vi "Test JSON Conversion.vi"() -> ()   [LabVIEW 2014]
uses:
  reusable/CRDS/Data/Cell/CRDS Cell Data.lvclass
  reusable/CRDS/Cell/extParam Ctl.ctl
  reusable/CRDS/Cell/hkParam Ctl.ctl
  reusable/PAS/Data/Cell/PAS Cell Data.lvclass
  reusable/CRDS/Data/Cell/CRDS Cell Data.lvclass/CRDS Cell Data.ctl
  reusable/PAS/Data/Cell/PAS Cell Data.lvclass/PAS Cell Data.ctl
  reusable/PAS/Data/Cell/Read fit data.vi
  reusable/PAS/Data/Cell/Read IAbackground.vi
  reusable/CRDS/Data/Cell/Read extParam.vi
  reusable/CRDS/Data/Cell/Read Allan Variances.vi
  reusable/PAS/Data/Cell/Read derived.vi
  reusable/PAS/Data/Cell/Read Fitted Data.vi
  reusable/PAS/Data/Cell/Read freqData.vi
  reusable/PAS/Data/Cell/Read timeData.vi
  reusable/PAS/Data/Cell/Read lasDiodeData.vi
  reusable/CRDS/Data/Cell/Read hkParam.vi
  reusable/CRDS/Data/Cell/Read Ringdowns.vi
  reusable/CRDS/CRDS Lib.lvlib
  <vilib>/measure/NI_MABase.lvlib
panel:
  out "Numeric Control":u32
  out "JSONData":string
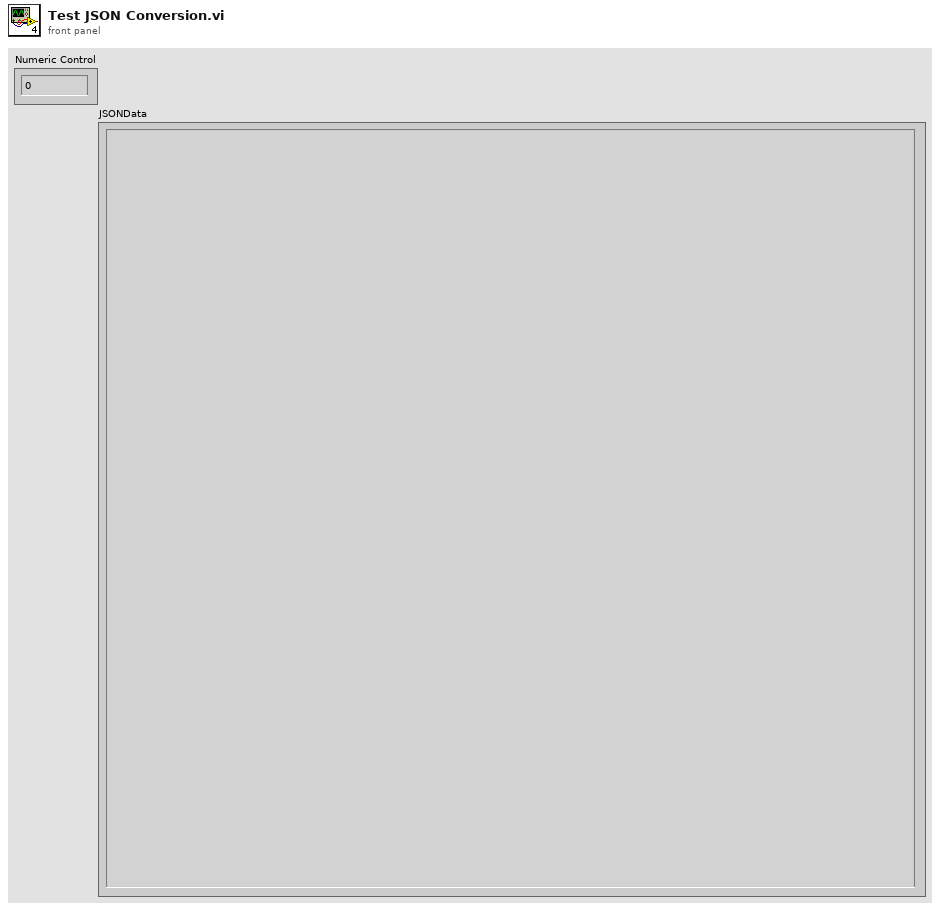
[diagram p1: front panel]
types:
  T1 = enum16{"Sine Wave", "Triangle Wave", "Square Wave", "Sawtooth Wave"}
  T2 = typedef "CRDS Lib.lvlib/extParam Ctl.ctl" = cluster{"Tau":sgl, "Tau0cor":sgl, "ext":sgl, "extCorr":sgl, "stdevTau":sgl, "eTau":sgl, "taucorr":sgl, "Tau0":sgl, "max":sgl}
  T3 = typedef "hkParam Ctl.ctl" = cluster{"rhDilFac":sgl, "Q":sgl, "Tmean":sgl, "extDilFac":sgl, "rhCell":sgl, "P":sgl, "T":sgl}
  T4 = cluster{"Time":dbl, "CellData":cluster{"extParam":T2, "hk":T3, "RDs":i16[][], "Data Access:Allan Variances":cluster{"iTime":sgl[], "stdev":sgl[]}}[]}
  T5 = cluster{"extParam":T2, "hk":T3, "RDs":i16[][], "Data Access:Allan Variances":cluster{"iTime":sgl[], "stdev":sgl[]}}
  T6 = typedef "extParam Ctl.ctl" = cluster{"Tau":sgl, "Tau0cor":sgl, "ext":sgl, "extCorr":sgl, "stdevTau":sgl, "eTau":sgl, "taucorr":sgl, "Tau0":sgl, "max":sgl}
  T7 = cluster{"f0":sgl, "IA":sgl, "Q":sgl, "max":dbl[], "noiseLim":dbl, "ext":dbl}
  T8 = typedef "NI_Matrix.lvlib/RealMatrix.ctl" = dbl[][]
  T9 = cluster{"Accessors:derived":cluster{"f0":sgl, "IA":sgl, "Q":sgl, "max":dbl[], "noiseLim":dbl, "ext":dbl}, "Accessors:fit data":cluster{"parameters":dbl[], "covariance":T8}, "Accessors:IAbackground":dbl}
  T10 = cluster{"extParam":T2, "hk":T3, "RDs":i16[][], "Data Access:Allan Variances":cluster{"iTime":sgl[], "stdev":sgl[]}}[]
  T11 = cluster{dbl, cluster{"Accessors:derived":cluster{"f0":sgl, "IA":sgl, "Q":sgl, "max":dbl[], "noiseLim":dbl, "ext":dbl}, "Accessors:fit data":cluster{"parameters":dbl[], "covariance":T8}, "Accessors:IAbackground":dbl}[], cluster{"Y":dbl[], "dt":dbl}[], cluster{"Y":dbl[], "dt":dbl}[], cluster{"Y":dbl[], "dt":dbl}[]}
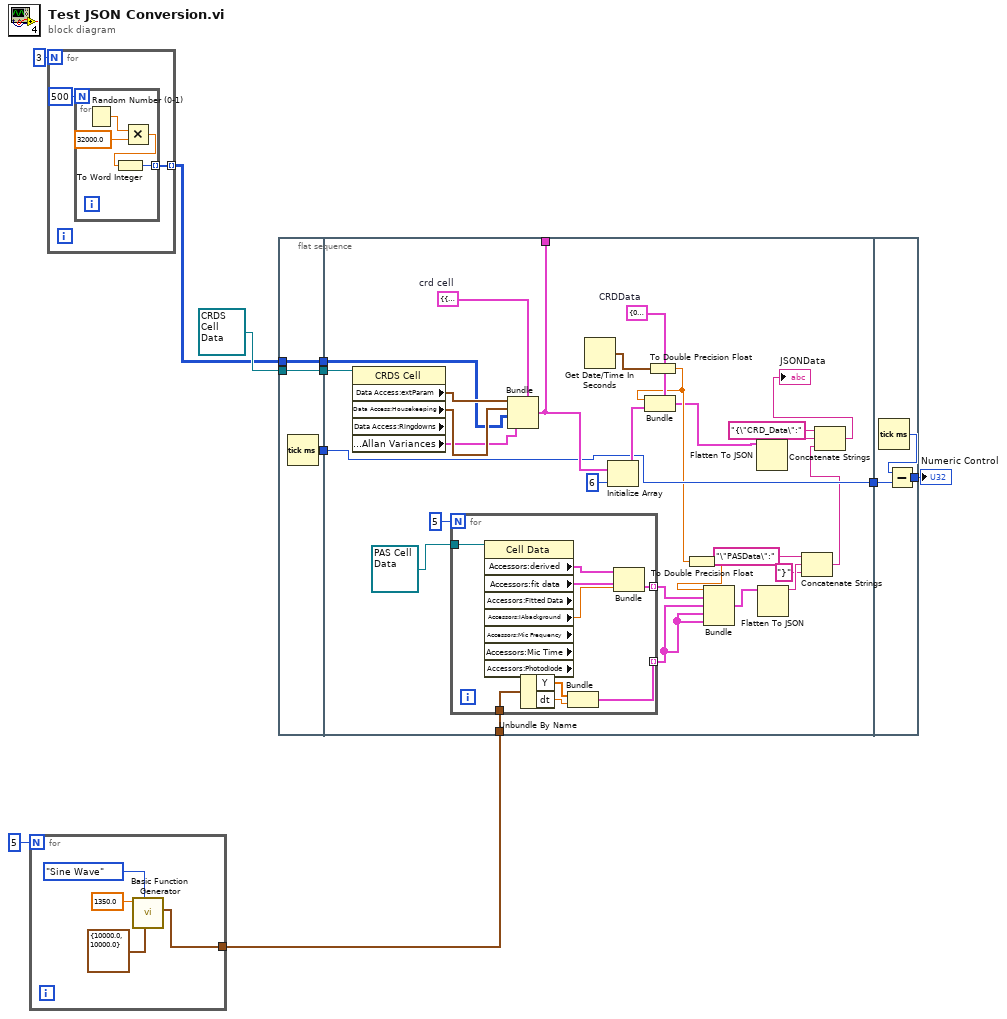
[diagram p0: block diagram]
diagram:
  n1 = for {
    N: 5 -> [_]
    tunnel: [w11] -> w1
    n2 = call <vilib>:"Basic Function Generator.vi"("sampling info"=cluster{"Fs":dbl, "#s":dbl} {"Fs"=10000.0, "#s"=10000.0}, "signal type"=T1."Sine Wave", "frequency"=1350.0) -> ("signal out"=w11:waveform(dbl))  [unwired: 6 in, 2 out]
  }
  n3 = for {
    N: 3 -> [_]
    tunnel: [w15] -> w8 mode=indexing
    n4 = for {
      N: 500 -> [_]
      tunnel: [w17] -> w15 mode=indexing
      n5 = Random Number (0-1)() -> (number: 0 to 1=w20:dbl)
      n6 = Multiply(x=w20, y=32000.0) -> (x*y=w18:dbl)
      n7 = To Word Integer(number=w18) -> (16bit integer=w17:i16)
    }
  }
  n8 = flat-sequence {
    tunnel: w8 -> [w22]
    tunnel: refnum<class "CRDS Cell Data.lvclass"> refnum ("CRDS Cell") -> [w23]
    tunnel: [w23] -> w7
    tunnel: [w22] -> w6
    tunnel: [w21] -> w4
    tunnel: [w45] -> _
    tunnel: w7 -> [w51]
    tunnel: w6 -> [w46]
    tunnel: [w41] -> w5
    tunnel: w4 -> [w41]
    tunnel: w1 -> [w36]
    tunnel: w5 -> [w62]
    tunnel: [w61] -> w3
    frame #0 {
      n9 = Tick Count (ms)() -> (millisecond timer value=w21:u32)
    }
    frame #1 {
      w40 = T4 {"Time"=0.0, "CellData"=[]}  # CRDData
      w47 = T5 {"extParam"={"Tau"=0.0, "Tau0cor"=0.0, "ext"=0.0, "extCorr"=0.0, "stdevTau"=0.0, "eTau"=0.0, "taucorr"=0.0, "Tau0"=0.0, "max"=0.0}, "hk"={"rhDilFac"=0.0, "Q"=0.0, "Tmean"=0.0, "extDilFac"=0.0, "rhCell"=0.0, "P"=0.0, "T"=0.0}, "RDs"=[], "Data Access:Allan Variances"={"iTime"=[], "stdev"=[]}}  # crd cell
      n10 = property class="CRDS Cell" props=["Data Access:extParam", "Data Access:Housekeeping", "Data Access:Ringdowns", "Data Access:Allan Variances"](reference=w51) -> ("Data Access:extParam"=w50:T6, "Data Access:Housekeeping"=w49:T3, "Data Access:Allan Variances"=w48:cluster{"iTime":i32[], sgl[]})  [unwired: 1 in, 3 out]
      n11 = for {
        N: 5 -> [_]
        tunnel: refnum<class "PAS Cell Data.lvclass"> refnum ("Cell Data") -> [w60]
        tunnel: w36 -> [w53]
        tunnel: [w56] -> w35 mode=indexing
        tunnel: [w52] -> w34 mode=indexing
        n12 = property class="Cell Data" props=["Accessors:derived", "Accessors:fit data", "Accessors:Fitted Data", "Accessors:IAbackground", "Accessors:Mic Frequency", "Accessors:Mic Time", "Accessors:Photodiode"](reference=w60) -> ("Accessors:derived"=w59:T7, "Accessors:fit data"=w58:cluster{"parameters":dbl[], "covariance":T8}, "Accessors:IAbackground"=w57:dbl)  [unwired: 1 in, 6 out]
        n13 = Unbundle By Name(w53) -> ("Y"=w54:dbl[], "dt"=w55:dbl)
        n14 = Bundle("Y"=w54, "dt"=w55) -> (w52:cluster{"Y":dbl[], "dt":dbl})  [unwired: 1 in]
        n15 = Bundle("Accessors:derived"=w59, "Accessors:fit data"=w58, "Accessors:IAbackground"=w57) -> (w56:T9)  [unwired: 1 in]
      }
      n16 = Bundle(cluster=w47, "extParam"=w50, "hk"=w49, "RDs"=w46, "Data Access:Allan Variances"=w48) -> (w45:T5)
      n17 = Get Date/Time In Seconds() -> (seconds since 1Jan1904=w43:timestamp)
      n18 = Initialize Array(w45, 6 ("dimension size")) -> (w42:T10)
      n19 = To Double Precision Float(number=w43) -> (double precision float=w38:dbl)
      n20 = Bundle(cluster=w40, "Time"=w38, "CellData"=w42) -> (w33:T4)
      n21 = To Double Precision Float(number=w38) -> (double precision float=w37:dbl)
      n22 = Bundle(w37, w35, w34, w34, w34) -> (w32:T11)  [unwired: 1 in]
      n23 = Flatten To JSON(anything=w33) -> (JSON string=w30:string)  [unwired: 2 in, 1 out]
      n24 = Flatten To JSON(anything=w32) -> (JSON string=w28:string)  [unwired: 2 in, 1 out]
      n25 = Concatenate Strings("\"PASData\":" ("string"), w28, "}" ("string")) -> (w25:string)
      n26 = Concatenate Strings("{\"CRD_Data\":" ("string"), w30, w25) -> (→"JSONData":string)
    }
    frame #2 {
      n27 = Tick Count (ms)() -> (millisecond timer value=w63:u32)
      n28 = Subtract(x=w63, y=w62) -> (x-y=w61:u32)
    }
  }
  "Numeric Control" <- w3
